vi "add_resonance_scanner_trigger.vi"(8 "Trigger":bool, 11 "Input":u32) -> (2 "Output":u32)   [LabVIEW 2012]
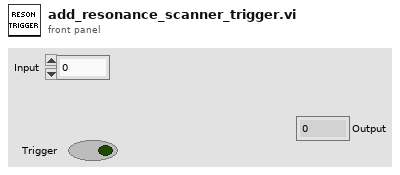
[diagram p1: front panel]
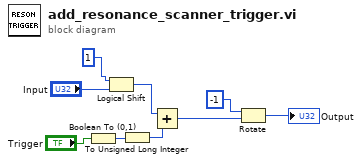
[diagram p0: block diagram]
diagram:
  n1 = Boolean To (0,1)(Boolean="Trigger") -> (0, 1=w2:i16)
  n2 = Logical Shift(y=i16 1, x="Input") -> (x << y=w4:u32)
  n3 = To Unsigned Long Integer(number=w2) -> (unsigned 32bit integer=w1:u32)
  n4 = Add(x=w4, y=w1) -> (x+y=w7:u32)
  n5 = Rotate(1:w7, 2:i16 -1) -> (0:→"Output":u32)
